vi "LED_MATRIX_GUI.vi"() -> ()   [LabVIEW 2023]
uses:
  <vilib>/Utility/miscctls.llb/LV3DPointTypeDef.ctl
  LabVIEW/Lab4_235/Serial - Settings.ctl
  <vilib>/Utility/miscctls.llb/LVRGBAColorTypeDef.ctl
  <vilib>/Analysis/coordinate.llb/3D Cartesian Coordinate Rotation (Euler) (Array).vi
  <vilib>/Instr/_visa.llb/VISA Configure Serial Port (Instr).vi
  <vilib>/picture/3D Picture Control/Object/Create Object (name).vi
  <vilib>/picture/3D Picture Control/Object/Add Object (no reference).vi
  <vilib>/picture/3D Picture Control/NI_3D Picture Control.lvlib
  <vilib>/Analysis/NI_AALPro.lvlib
panel:
  in  "Euler Angles":cluster{"Roll":dbl, "Pitch":dbl, "Yaw":dbl}
  out "After Roll":string
  in  "Roll":dbl(slide) scale=0.0..360.0
  in  "X 2":bool
  in  "X":bool
  in  "Z_down":bool
  in  "Z":bool
  in  "Y_down":bool
  in  "Y":bool
  in  "X_down":bool
  in  "X":bool
  out "Numeric":i32
  out "Input Coordinates":string
  in  "Axis label?":bool
  out "Read Buffer":string
  in  "Serial Settings":T1={"baud rate"=115200, "data bits"=8, "parity"=enum."None", "stop bits"=10, "flow control"=0} {"flow control" items=["None"=0, "XON/XOFF"=1, "RTS/CTS"=2, "DTR/DSR"=4]; "stop bits" items=["1.0"=10, "1.5"=15, "2.0"=20]; "data bits" min=5 max=8 step=1; "baud rate" items=["75"=75, "110"=110, "134"=134, "150"=150, "300"=300, "600"=600, "1200"=1200, "1800"=1800, "2400"=2400, "4800"=4800, "7200"=7200, "9600"=9600, "14400"=14400, "19200"=19200, "28800"=28800, "38400"=38400, "56000"=56000, "57600"=57600, "115200"=115200, "128000"=128000, "230400"=230400]}
  in  "VISA resource name":refnum<visa-resource-name>
  in  "Up Direction":T2
  in  "Target":T2
  in  "Camera Position":T2
  in  "File path (dialog if empty)":path
  in  "From File?":bool
  in  "Camera Controller:":T3(ring)=enum."Spherical"
  in  "stop":bool
  out "3D Picture":refnum<vi>(3d-picture)
  # "Overview:  Code that shows how to load a 3D point cloud data into a 3D picture control in LabVIEW.\nRequirements: LabVIEW 2012 or compatible\nInstructions:\n1. Select if you would like to load from file or generate a random object.\n2. Run the VI.\n3. Use the Camera Controller to adjust the way the mouse moves the 3D object.\n4. Press ESC button to stop."
  # "Translation"
  # "Rotation"
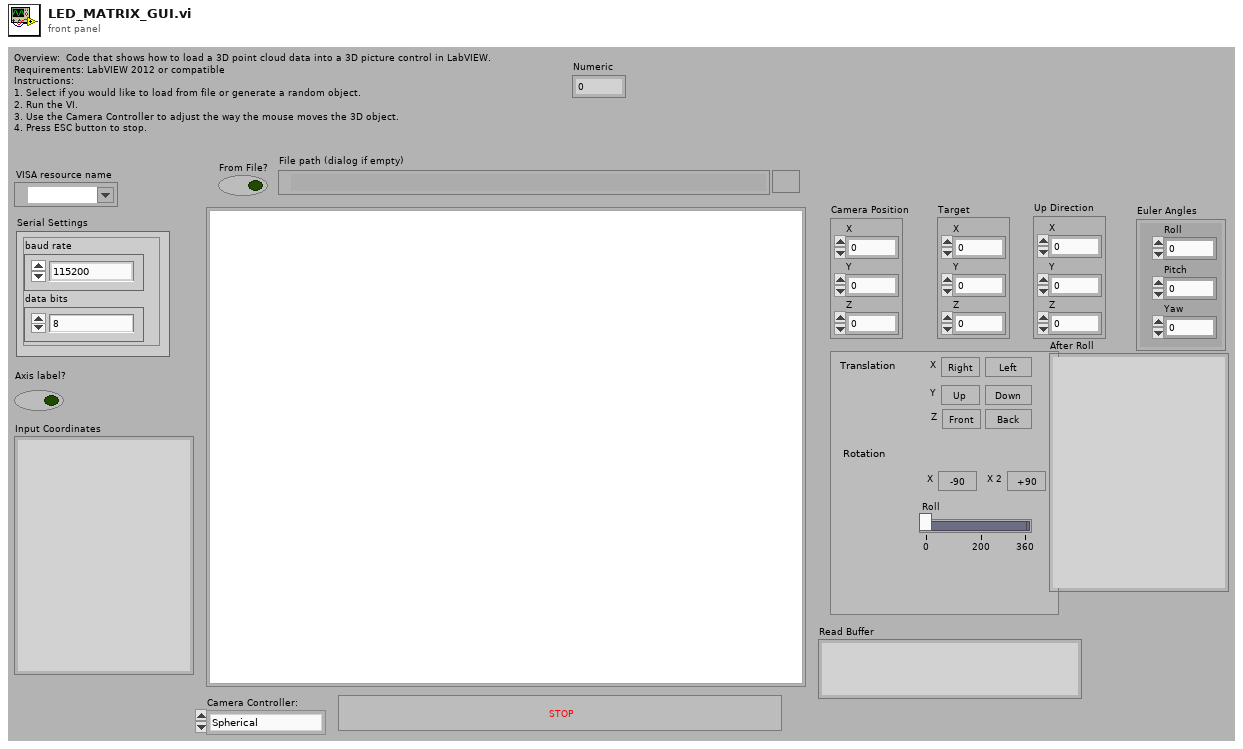
[diagram p1: front panel]
types:
  T1 = typedef "Serial - Settings.ctl" = cluster{"baud rate":u32, "data bits":u16, "parity":enum16{"None", "Odd", "Even", "Mark", "Space"}, "stop bits":u16, "flow control":u16}
  T2 = typedef "LV3DPointTypeDef.ctl" = cluster{"X":sgl, "Y":sgl, "Z":sgl}
  T3 = enum16{"None", "Spherical", "Flying", "Oriented"}
  T4 = typedef "LVRGBAColorTypeDef.ctl" = cluster{"Red":sgl, "Green":sgl, "Blue":sgl, "Alpha":sgl}
  T5 = enum16{"Overall", "Per Primitive", "Per Vertex", "Binding Off"}
  T6 = enum16{"Points", "Lines", "Line Strip", "Line Loop", "Triangles", "Triangle Strip", "Triangle Fan", "Quads", "Quad Strip", "Polygon"}
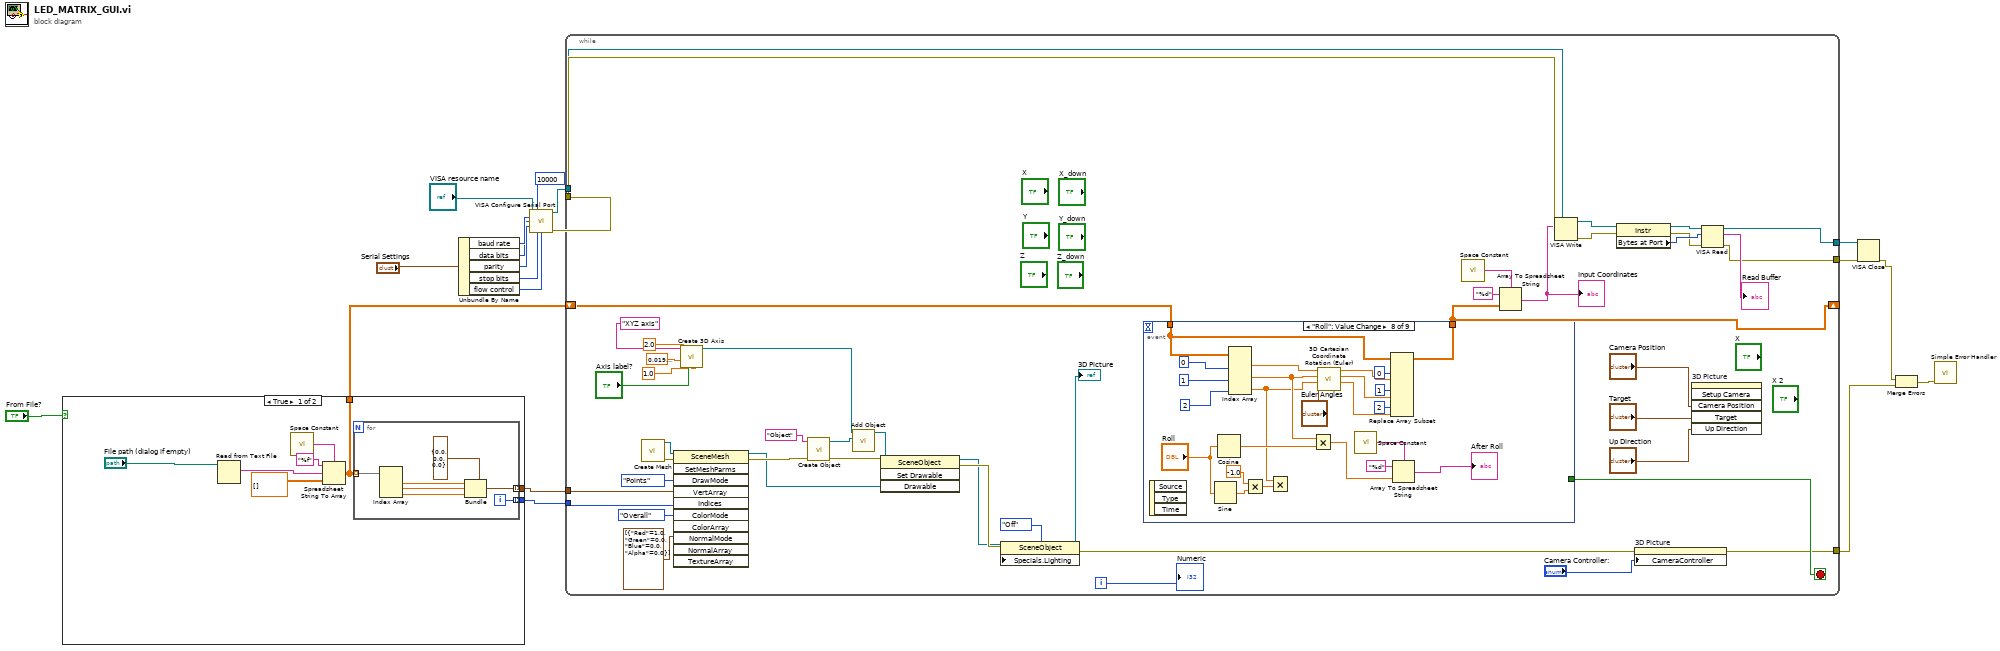
[diagram p0: block diagram]
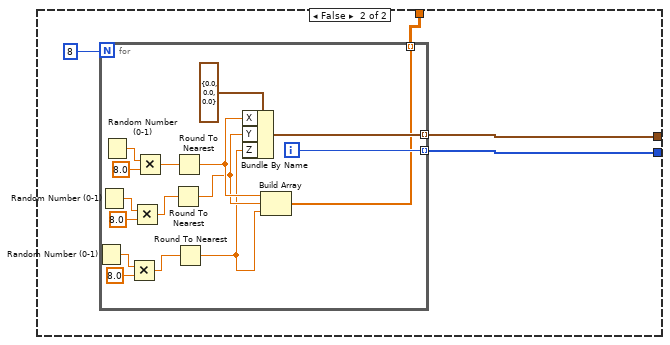
[diagram p2: hidden frame]
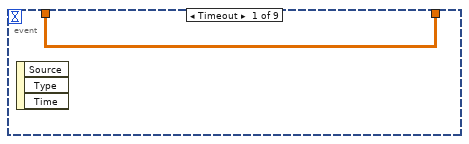
[diagram p3: hidden frame]
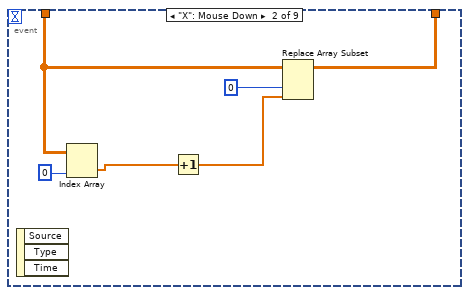
[diagram p4: hidden frame]
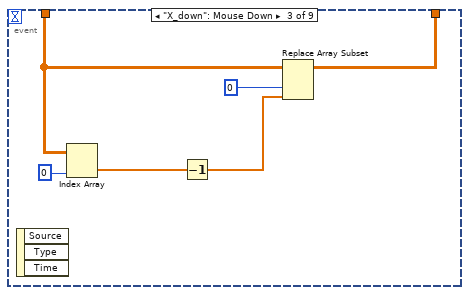
[diagram p5: hidden frame]
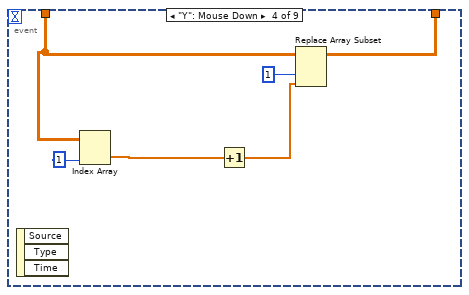
[diagram p6: hidden frame]
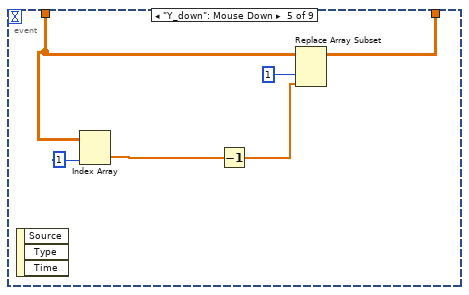
[diagram p7: hidden frame]
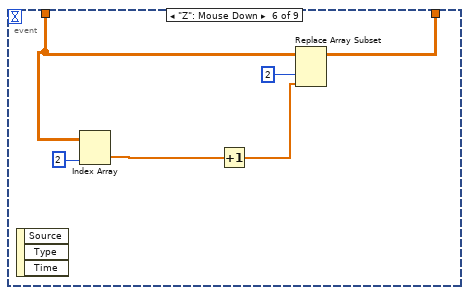
[diagram p8: hidden frame]
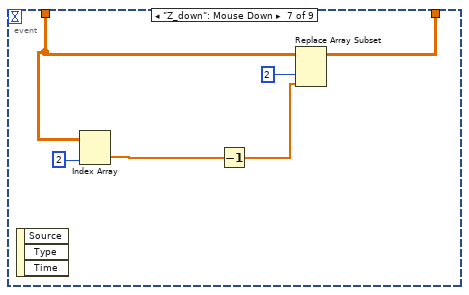
[diagram p9: hidden frame]
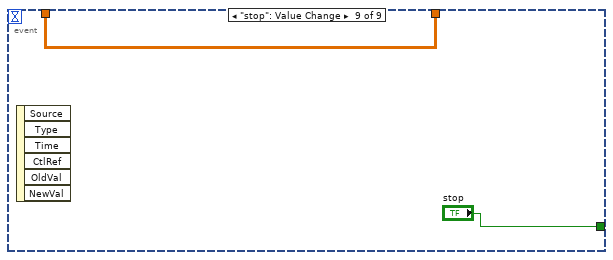
[diagram p10: hidden frame]
diagram:
  n1 = case shown="True" "From File?" {
    tunnel: [w22 w37] -> w6
    tunnel: [w21 w36] -> w5
    tunnel: [w20 w35] -> w1
    frame True {
      n2 = Read from Text File(file (use dialog)="File path (dialog if empty)") -> (text=w26:string)  [unwired: 3 in, 3 out]
      n3 = call <vilib>:"Space Constant.vi"() -> ("String"=w25:string)
      n4 = Spreadsheet String To Array(delimiter (Tab)=w25, format string="%f", spreadsheet string=w26, array type (2D Dbl)=sgl[][] []) -> (array=w20:sgl[][])
      n5 = for {
        tunnel: w20 -> [w34] mode=indexing
        tunnel: [w29] -> w22 mode=indexing
        tunnel: [w28] -> w21 mode=indexing
        i -> [w28]
        n6 = Index Array(array=w34) -> (element #1=w32:sgl, element #2=w31:sgl, element #3=w30:sgl)  [unwired: 3 in]
        n7 = Bundle(cluster=T2 {"X"=0.0, "Y"=0.0, "Z"=0.0} ("3D Point"), "X"=w32, "Y"=w31, "Z"=w30) -> (w29:T2)
      }
    }
    frame False {
      n8 = for {
        N: 8 -> [_]
        tunnel: [w47] -> w37 mode=indexing
        tunnel: [w46] -> w36 mode=indexing
        tunnel: [w45] -> w35 mode=indexing
        i -> [w46]
        n9 = Random Number (0-1)() -> (number: 0 to 1=w48:dbl)
        n10 = Random Number (0-1)() -> (number: 0 to 1=w51:dbl)
        n11 = Random Number (0-1)() -> (number: 0 to 1=w52:dbl)
        n12 = Multiply(x=w48, y=8.0) -> (x*y=w40:dbl)
        n13 = Multiply(x=w51, y=8.0) -> (x*y=w42:dbl)
        n14 = Multiply(x=w52, y=8.0) -> (x*y=w44:dbl)
        n15 = Round To Nearest(number=w42) -> (nearest integer value=w41:dbl)
        n16 = Round To Nearest(number=w44) -> (nearest integer value=w43:dbl)
        n17 = Round To Nearest(number=w40) -> (nearest integer value=w39:dbl)
        n18 = Bundle By Name(cluster=T2 {"X"=0.0, "Y"=0.0, "Z"=0.0} ("3D Point"), "X"=w43, "Y"=w41, "Z"=w39) -> (w47:T2)
        n19 = Build Array(w43, w41, w39) -> (w45:dbl[])
      }
    }
  }
  n20 = Unbundle By Name("Serial Settings") -> ("baud rate"=w16:u32, "data bits"=w15:u16, "parity"=w14:enum16{"None", "Odd", "Even", "Mark", "Space"}, "stop bits"=w13:u16, "flow control"=w12:u16)
  n21 = call-poly "VISA Configure Serial Port"("VISA resource name"="VISA resource name", "timeout (10sec)"=u32 10000, "baud rate (9600)"=w16, "data bits (8)"=w15, "parity (0:none)"=w14, "stop bits (10: 1 bit)"=w13, "flow control (0:none)"=w12) -> ("VISA resource name out"=w9:refnum<visa-resource-name>, "error out"=w10:errorcluster)  [unwired: 7 in]
  n22 = while {
    tunnel: w10 -> [w93]
    tunnel: w9 -> [w92]
    tunnel: [w91] -> w8
    tunnel: [w90] -> w7
    tunnel: w6 -> [w63]
    tunnel: w5 -> [w62]
    tunnel: [w57] -> w3
    shift-right: [w55] -> _
    shift-left: w1 -> [w82]
    i -> [w81]
    stop <- w83 stop-if-true
    n23 = call <vilib>:"Create Mesh.vi"() -> ("error out"=w74:errorcluster, "New Mesh Refnum"=w71:refnum<vi>)  [unwired: 10 in]
    n24 = invoke class="SceneMesh" method="SetMeshParms"(reference=w71, error in=w74, "DrawMode"=T6."Points" ("Draw Mode"), "VertArray"=w63, "Indices"=w62, "ColorMode"=T5."Overall" ("Color Binding Mode"), "ColorArray"=T4[] [{"Red"=1.0, "Green"=0.0, "Blue"=0.0, "Alpha"=0.0}] ("Color Array")) -> (reference out=w72:refnum<vi>, error out=w76:errorcluster)  [unwired: 4 in, 9 out]
    n25 = call <vilib>:"Create 3D Axis.vi"("Character Size"=sgl 1.0, "Axis label?"="Axis label?", "Radius"=sgl 0.02, "Length"=sgl 2.0, "Name"="XYZ axis") -> ("New Object Refnum"=w78:refnum<vi>)  [unwired: 5 in, 1 out]
    n26 = call-poly <vilib>:"Create Object.vi"("error in (no error)"=w76, "Name"="Object") -> ("error out"=w77:errorcluster, "Scene:New Object"=w79:refnum<vi>)  [unwired: 8 in]
    n27 = call-poly <vilib>:"Add Object.vi"("New Object In"=w79, "Scene Object In"=w78) -> ("Scene Object Out"=w56:refnum<vi>)  [unwired: 8 in, 1 out]
    n28 = invoke class="SceneObject" method="Set Drawable"(reference=w56, error in=w77, "Drawable"=w72) -> (reference out=w73:refnum<vi>, error out=w75:errorcluster)  [unwired: 1 in, 2 out]
    n29 = property class="SceneObject"(reference=w73, error in=w75, "Specials.Lighting"=enum16{"Inherit Value", "Off", "On"}."Off" ("Specials:Lighting")) -> (reference out=→"3D Picture":refnum<vi>, error out=w58:errorcluster)
    n30 = event shown="[7] \"Roll\": Value Change" {
      selector: _ -> [_ _ _ _ _ _ _ _ _]
      dyn-events: _ -> [_ _ _ _ _ _ _ _ _]
      timeout: _ -> [_ _ _ _ _ _ _ _ _]
      tunnel: [_ _ _ _ _ _ _ _ "stop"] -> w83
      tunnel: w82 -> [w101 w106 w112 w117 w123 w129 w135 w154 w162]
      tunnel: [w101 w104 w110 w116 w122 w128 w134 w158 w162] -> w55
      event Timeout {
        n31 = event-data() -> ()  [unwired: 1 in, 3 out]
      }
      event "X": Mouse Down {
        n32 = event-data() -> ()  [unwired: 1 in, 3 out]
        n33 = Index Array "Index Array"(array=w106, index (col)=0 ("disabled index (col)")) -> (element=w103:dbl[])  [unwired: 1 in]
        n34 = Increment(x=w103) -> (x+1=w102:dbl[])
        n35 = Replace Array Subset(array=w106, new element=w102, index (col)=0 ("disabled index (col)")) -> (w104:dbl[][])  [unwired: 1 in]
      }
      event "X_down": Mouse Down {
        n36 = event-data() -> ()  [unwired: 1 in, 3 out]
        n37 = Index Array "Index Array"(array=w112, index (col)=0 ("disabled index (col)")) -> (element=w109:dbl[])  [unwired: 1 in]
        n38 = Decrement(x=w109) -> (x-1=w108:dbl[])
        n39 = Replace Array Subset(array=w112, new element=w108, index (col)=0 ("disabled index (col)")) -> (w110:dbl[][])  [unwired: 1 in]
      }
      event "Y": Mouse Down {
        n40 = event-data() -> ()  [unwired: 1 in, 3 out]
        n41 = Index Array "Index Array"(array=w117, index (col)=1 ("disabled index (col)")) -> (element=w114:dbl[])  [unwired: 1 in]
        n42 = Increment(x=w114) -> (x+1=w115:dbl[])
        n43 = Replace Array Subset "Replace Array Subset"(array=w117, new element=w115, index (col)=1 ("disabled index (col)")) -> (w116:dbl[][])  [unwired: 1 in]
      }
      event "Y_down": Mouse Down {
        n44 = event-data() -> ()  [unwired: 1 in, 3 out]
        n45 = Index Array "Index Array"(array=w123, index (col)=1 ("disabled index (col)")) -> (element=w120:dbl[])  [unwired: 1 in]
        n46 = Decrement(x=w120) -> (x-1=w121:dbl[])
        n47 = Replace Array Subset "Replace Array Subset"(array=w123, new element=w121, index (col)=1 ("disabled index (col)")) -> (w122:dbl[][])  [unwired: 1 in]
      }
      event "Z": Mouse Down {
        n48 = event-data() -> ()  [unwired: 1 in, 3 out]
        n49 = Index Array "Index Array"(array=w129, index (col)=2 ("disabled index (col)")) -> (element=w126:dbl[])  [unwired: 1 in]
        n50 = Increment(x=w126) -> (x+1=w127:dbl[])
        n51 = Replace Array Subset "Replace Array Subset"(array=w129, new element=w127, index (col)=2 ("disabled index (col)")) -> (w128:dbl[][])  [unwired: 1 in]
      }
      event "Z_down": Mouse Down {
        n52 = event-data() -> ()  [unwired: 1 in, 3 out]
        n53 = Index Array "Index Array"(array=w135, index (col)=2 ("disabled index (col)")) -> (element=w132:dbl[])  [unwired: 1 in]
        n54 = Decrement(x=w132) -> (x-1=w133:dbl[])
        n55 = Replace Array Subset "Replace Array Subset"(array=w135, new element=w133, index (col)=2 ("disabled index (col)")) -> (w134:dbl[][])  [unwired: 1 in]
      }
      event "Roll": Value Change {
        n56 = event-data() -> ()  [unwired: 1 in, 3 out]
        n57 = Sine(x="Roll") -> (sin(x)=w146:dbl)
        n58 = Cosine(x="Roll") -> (cos(x)=w152:dbl)
        n59 = Index Array(array=w154, index (col) #1=0 ("disabled index (col)"), index (col) #2=1 ("index (col)"), index (col) #3=2 ("index (col)")) -> (element #1=w144:dbl[], element #2=w143:dbl[], element #3=w142:dbl[])  [unwired: 3 in]
        n60 = Multiply(x=-1.0, y=w146) -> (x*y=w147:dbl)
        n61 = Multiply(x=w142, y=w147) -> ()  [unwired: 1 out]
        n62 = Multiply(x=w143, y=w152) -> (x*y=w148:dbl[])
        n63 = call-poly <vilib>:"3D Cartesian Coordinate Rotation (Euler).vi"("Euler Angles"="Euler Angles", "Z"=w142, "Y"=w143, "X"=w144) -> ("Z Out"=w139:dbl[], "Y Out"=w140:dbl[], "X Out"=w141:dbl[])  [unwired: 4 in, 1 out]
        n64 = call <vilib>:"Space Constant.vi"() -> ("String"=w149:string)
        n65 = Replace Array Subset(array=w154, new element #1=w141, index (col) #1=0 ("index (col)"), new element #2=w140, index (col) #2=1 ("index (col)"), new element #3=w139, index (col) #3=2 ("index (col)")) -> (w158:dbl[][])  [unwired: 3 in]
        n66 = Array To Spreadsheet String(delimiter (Tab)=w149, array=w148, 3:"%d" ("format string")) -> (spreadsheet string=→"After Roll":string)
      }
      event "stop": Value Change {
        n67 = event-data() -> ()  [unwired: 1 in, 6 out]
      }
    }
    n68 = call <vilib>:"Space Constant.vi"() -> ("String"=w87:string)
    n69 = Array To Spreadsheet String(delimiter (Tab)=w87, array=w55, 3:"%d" ("format string")) -> (spreadsheet string=w89:string)
    "Input Coordinates" <- w89
    n70 = VISA Write(VISA resource name=w92, write buffer=w89, error in (no error)=w93) -> (VISA resource name out=w95:refnum<visa-resource-name>, error out=w97:errorcluster)  [unwired: 1 out]
    n71 = property on="Property Node" class="Instr"(reference=w95, error in=w97) -> (reference out=w96:refnum<visa-resource-name>, error out=w98:errorcluster, "Bytes at Port"=w99:u32)
    n72 = property on="3D Picture" class="SceneGraphDisp (strict)"(error in=w58, "CameraController"="Camera Controller:") -> (error out=w57:errorcluster)  [unwired: 1 in, 1 out]
    n73 = invoke on="3D Picture" class="SceneGraphDisp (strict)" method="Setup Camera"("Camera Position"="Camera Position", "Target"="Target", "Up Direction"="Up Direction") -> ()  [unwired: 3 in, 6 out]
    n74 = VISA Read(VISA resource name=w96, byte count=w99, error in (no error)=w98) -> (VISA resource name out=w91:refnum<visa-resource-name>, read buffer=→"Read Buffer":string, error out=w90:errorcluster)  [unwired: 1 out]
    "Numeric" <- w81
  }
  n75 = VISA Close(VISA resource name=w8, error in (no error)=w7) -> (error out=w4:errorcluster)
  n76 = Merge Errors(w4, w3) -> (w2:errorcluster)
  n77 = call <vilib>:"Simple Error Handler.vi"("error in (no error)"=w2) -> ()  [unwired: 4 in, 5 out]
